vi "VoltageScan.vi"() -> ()   [LabVIEW 2015]
uses:
  Program Files (x86)/National Instruments/LabVIEW 2016/instr.lib/Agilent 428X Series/Agilent 428X Series.lvlib
  Program Files (x86)/National Instruments/LabVIEW 2016/instr.lib/Keithley 24XX/Keithley 24XX.lvlib
  <vilib>/Utility/file.llb/Write Delimited Spreadsheet (string).vi
  <vilib>/Utility/file.llb/Read Delimited Spreadsheet (DBL).vi
  Program Files (x86)/National Instruments/LabVIEW 2016/instr.lib/Keithley 24XX/Public/Data/Read (Single Point).vi
panel:
  in  "Display channel":i32
  out "Data curve for single channel":cluster{"X":dbl[], "Y":dbl[]}[](graph) caption="XY Graph"
  in  "Voltage Limit (V)":dbl=1000.0 format="%#_13g"
  in  "Stop":bool
  in  "Sensor type":enum16{"6''", "8''", "One channel"}(ring)=enum."One channel"
  out "Channels":cluster{i32[], dbl[]}[](graph) caption="XY Graph"
  in  "Voltage Delay (s)":dbl=0.5 format="%#_13g"
  out "Data Status":bool=TRUE
  in  "VISA resource name LCR":refnum<visa-resource-name>
  in  "Compliance  Level (uA)":dbl=10.0
  in  "Enable Voltage Auto Range (T:Enable)":bool=TRUE
  in  "Voltage Manual Range (1.0)":dbl=1.0
  in  "VISA resource name":refnum<visa-resource-name>
  in  "Open after execution?":bool
  out "Output file":path
  in  "Output file":string="test.txt"
  out "Current voltage [V]":dbl
  out "Current channel":i32
  in  "Switch Delay (s)":dbl=0.01 format="%#_13g"
  out "Voltages":cluster{"X":dbl[], "Y":dbl[]}[](graph) caption="XY Graph"
  out "Input file":path
  in  "Measurement type":enum16{"IV", "CV", "Test"}(ring)=enum."Test"
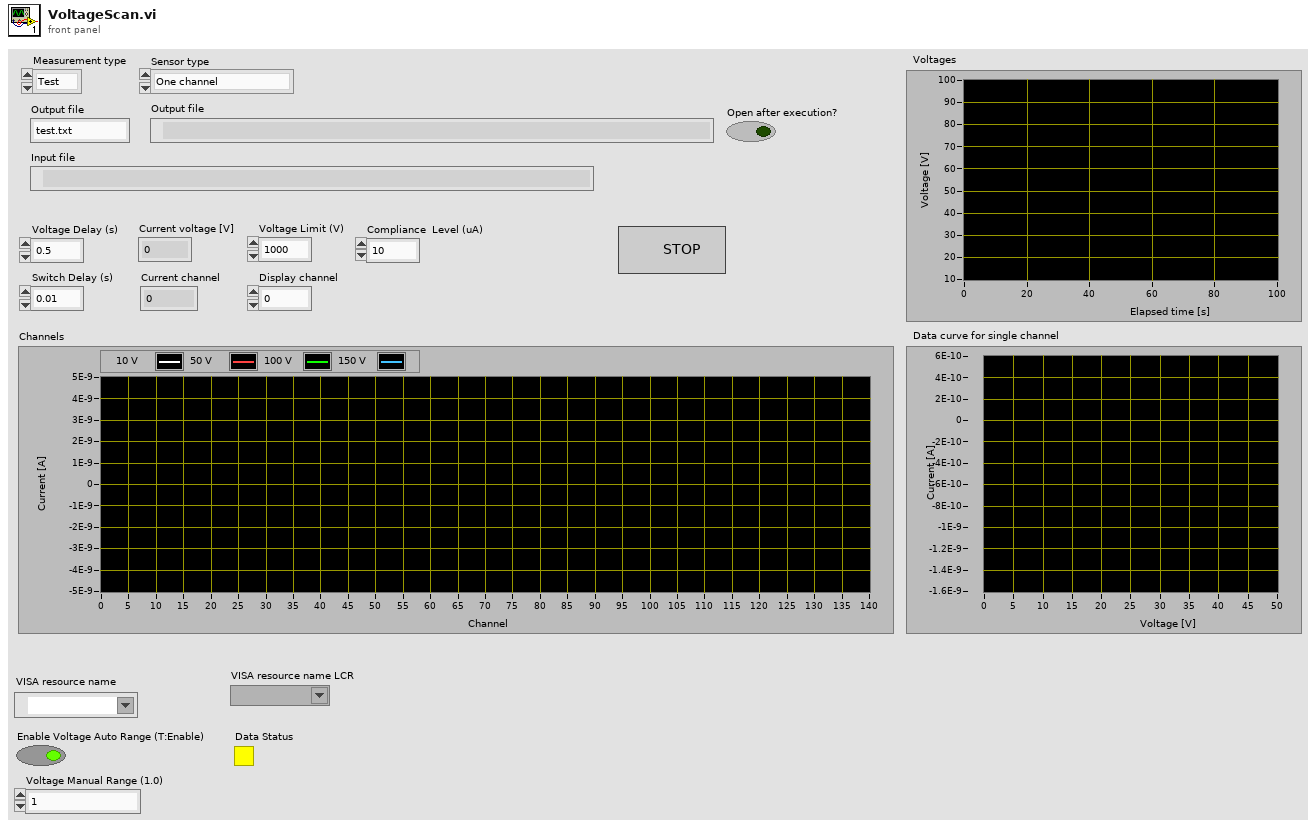
[diagram p1: front panel]
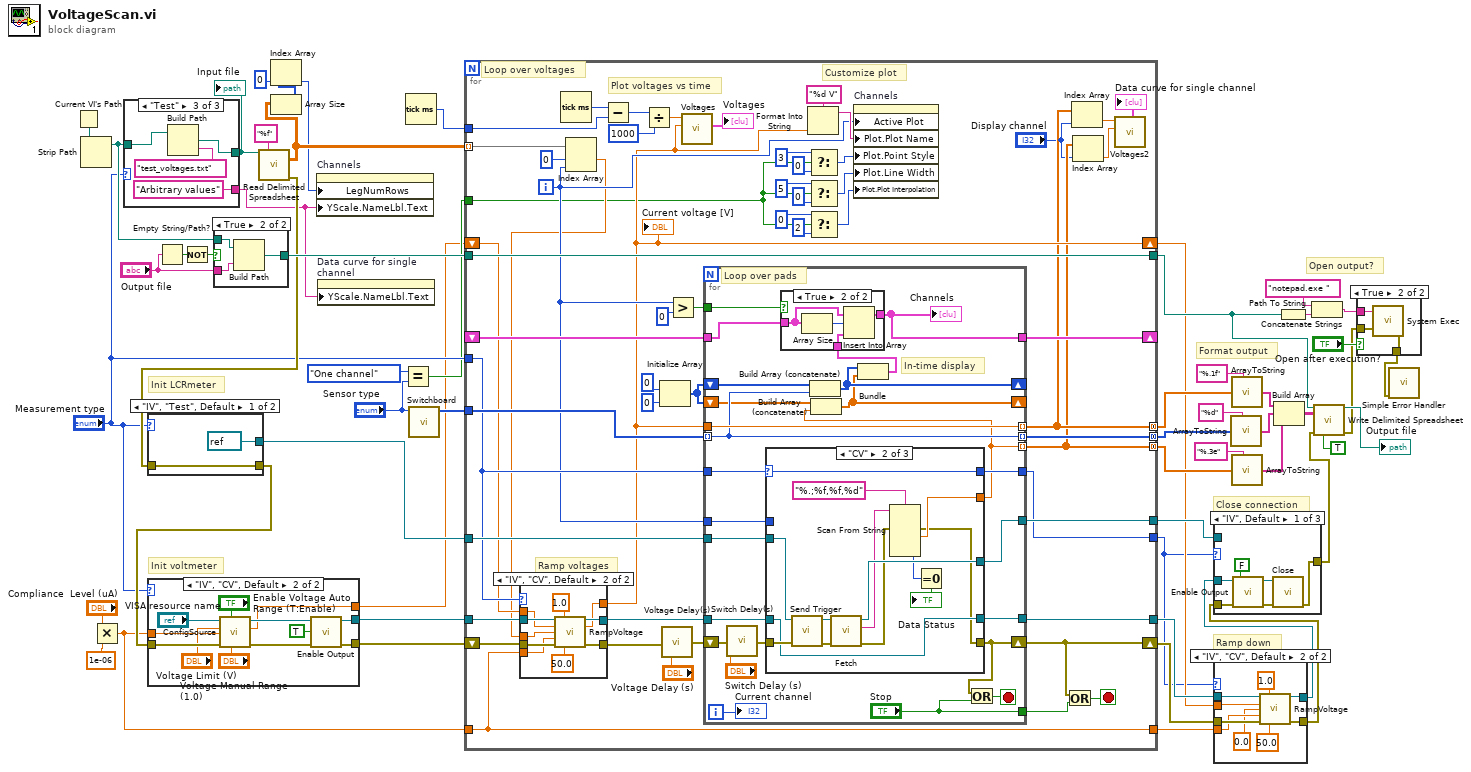
[diagram p0: block diagram]
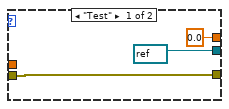
[diagram p3: hidden frame]
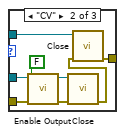
[diagram p4: hidden frame]
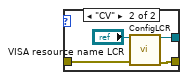
[diagram p6: hidden frame]
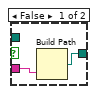
[diagram p8: hidden frame]
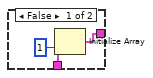
[diagram p10: hidden frame]
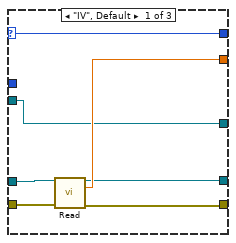
[diagram p11: hidden frame]
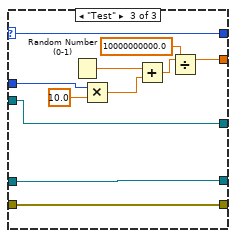
[diagram p12: hidden frame]
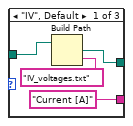
[diagram p13: hidden frame]
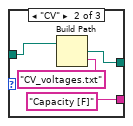
[diagram p14: hidden frame]
diagram:
  # "Close connection"
  # "Ramp down"
  # "Init LCRmeter"
  # "Init voltmeter"
  # "Format output"
  # "Open output?"
  n1 = Current VI's Path() -> (path=w55:path)
  n2 = Strip Path(path=w55) -> (stripped path=w49:path)  [unwired: 1 out]
  n3 = Multiply(x="Compliance  Level (uA)", y=1e-06) -> (x*y=w5:dbl)
  n4 = case shown="\"Test\"" "Measurement type" {
    tunnel: [w58 w62 w66] -> w30
    tunnel: w49 -> [w60 w63 w67]
    tunnel: ["Current [A]" "Capacity [F]" "Arbitrary values"] -> w2
    frame "IV", Default {
      n5 = Build Path(base path=w60, name or relative path="IV_voltages.txt") -> (appended path=w58:path)
    }
    frame "CV" {
      n6 = Build Path(base path=w63, name or relative path="CV_voltages.txt") -> (appended path=w62:path)
    }
    frame "Test" {
      n7 = Build Path(base path=w67, name or relative path="test_voltages.txt") -> (appended path=w66:path)
    }
  }
  "Input file" <- w30
  n8 = Empty String/Path?(string/path="Output file") -> (empty?=w47:bool)
  n9 = Not(x=w47) -> (.not. x?=w45:bool)
  n10 = case shown="True" w45 {
    tunnel: "Output file" -> [w70 w73]
    tunnel: w49 -> [_ w72]
    tunnel: [w69 w71] -> w28
    frame False {
      n11 = Build Path(name or relative path=w70) -> (appended path=w69:path)  [unwired: 1 in]
    }
    frame True {
      n12 = Build Path(base path=w72, name or relative path=w73) -> (appended path=w71:path)
    }
  }
  n13 = call-poly <vilib>:"Read Delimited Spreadsheet.vi"("file path (dialog if empty)"=w30, "format (%.3f)"="%f") -> ("all rows"=w52:dbl[][], "error out"=w24:errorcluster)  [unwired: 8 in, 4 out]
  n14 = case shown="\"IV\", \"Test\", Default" "Measurement type" {
    tunnel: w24 -> [w75 w78]
    tunnel: [w75 w77] -> w23
    tunnel: [refnum<visa-resource-name> refnum ("VISA resource name out") w76] -> w22
    frame "IV", "Test", Default {
    }
    frame "CV" {
      n15 = call "ConfigLCR.vi"("VISA resource name LCR"="VISA resource name LCR", "error in (no error)"=w78) -> ("VISA resource name out"=w76:refnum<visa-resource-name>, "error out"=w77:errorcluster)  [unwired: 12 in]
    }
  }
  n16 = case shown="\"IV\", \"CV\", Default" "Measurement type" {
    tunnel: [refnum<visa-resource-name> refnum ("VISA resource name out") w93] -> w27
    tunnel: [w82 w92] -> w26
    tunnel: w23 -> [w82 w87]
    tunnel: w5 -> [_ w84]
    tunnel: [0.0 ("Output Level (0)") w83] -> w11
    frame "Test" {
    }
    frame "IV", "CV", Default {
      n17 = call "ConfigSource.vi"("Voltage Manual Range (1.0)"="Voltage Manual Range (1.0)", "Single measurement? 2"="Enable Voltage Auto Range (T:Enable)", "error in (no error)"=w87, "Compliance  Level (0.1)"=w84, "Voltage Limit (0.0 V)"="Voltage Limit (V)", "VISA resource name"="VISA resource name") -> ("error out"=w90:errorcluster, "Output Level (0)"=w83:dbl, "VISA resource name out"=w91:refnum<visa-resource-name>)  [unwired: 3 in]
      n18 = call "Enable Output.vi"("error in (no error)"=w90, "Enable Output (T: Enable)"=TRUE ("Enable Output"), "VISA resource name"=w91) -> ("error out"=w92:errorcluster, "VISA resource name out"=w93:refnum<visa-resource-name>)  [unwired: 7 in]
    }
  }
  n19 = Array Size(array=w52) -> (size(s)=w54:i32[])
  n20 = Index Array(array=w54, index=0) -> (element=w17:i32)
  n21 = property on="Channels" class="XYGraph (strict)"("LegNumRows"=w17, "YScale.NameLbl.Text"=w2) -> ()  [unwired: 2 in, 2 out]
  n22 = property on="Data curve for single channel" class="XYGraph (strict)"("YScale.NameLbl.Text"=w2) -> ()  [unwired: 2 in, 2 out]
  n23 = Equal?(x=enum16{"6''", "8''", "One channel"}."One channel" ("Sensor type 2"), y="Sensor type") -> (x = y?=w14:bool)
  n24 = Tick Count (ms)() -> (millisecond timer value=w18:u32)
  n25 = call "Switchboard.vi"("Sensor type"="Sensor type") -> ("Output config"=w51:i32[])  [unwired: 10 in]
  n26 = for {
    tunnel: w52 -> [w149] mode=indexing
    tunnel: w51 -> [w146]
    tunnel: [w101] -> w37 mode=concatenating
    tunnel: [w100] -> w35 mode=concatenating
    tunnel: [w144] -> w36 mode=concatenating
    tunnel: w28 -> [w143]
    tunnel: [w143] -> w25
    tunnel: w27 -> [w142]
    tunnel: [w107] -> w7
    tunnel: "Measurement type" -> [w120]
    shift-right: [w106] -> w8
    shift-left: w26 -> [w139]
    tunnel: w22 -> [w138]
    tunnel: [w134] -> w3
    tunnel: [w140] -> w21
    shift-right: [w132] -> _
    shift-left: _ -> [w131]
    tunnel: w18 -> [w125]
    tunnel: w14 -> [w95]
    tunnel: w5 -> [w104]
    shift-right: [w102] -> w6
    shift-left: w11 -> [w105]
    tunnel: [w104] -> w4
    i -> [w110]
    stop <- w108 stop-if-true
    # "Ramp voltages"
    # "Plot voltages vs time"
    # "Customize plot"
    # "Loop over voltages"
    n27 = Tick Count (ms)() -> (millisecond timer value=w127:u32)
    n28 = Index Array(array=w149, index #1=0 ("index"), index #2=w110) -> (element #1=w103:dbl)  [unwired: 1 out]
    n29 = case shown="\"IV\", \"CV\", Default" w120 {
      tunnel: w142 -> [w152 w159]
      tunnel: w103 -> [w150 w158]
      tunnel: [w152 w161] -> w141
      tunnel: w139 -> [w151 w160]
      tunnel: [w151 w162] -> w136
      tunnel: w104 -> [_ w156]
      tunnel: w105 -> [_ w157]
      tunnel: [w150 w153] -> w102
      frame "Test" {
      }
      frame "IV", "CV", Default {
        n30 = call "RampVoltage.vi"("VISA resource name"=w159, "Delay (s)"=1.0, "Current voltage (V)"=w157, "Target voltage (V)"=w158, "Compliance Current (A)"=w156, "error in (no error)"=w160, "Step size (V)"=50.0) -> ("VISA resource name out"=w161:refnum<visa-resource-name>, "Current voltage out (V)"=w153:dbl, "error out"=w162:errorcluster)  [unwired: 6 in]
      }
    }
    "Current voltage [V]" <- w102
    n31 = Subtract(x=w127, y=w125) -> (x-y=w126:u32)
    n32 = Divide(x=w126, y=u32 1000 ("x")) -> (x/y=w124:dbl)
    n33 = Initialize Array(0 ("dimension size"), 0 ("dimension size")) -> (w128:i32[])
    n34 = call "Voltage Delay(s)"("error in (no error)"=w136, "Delay Time (s)"="Voltage Delay (s)") -> ("error out"=w135:errorcluster)  [unwired: 9 in]
    n35 = Greater?(x=w110, y=0) -> (0:w133:bool)
    n36 = call "Voltages"("Y Input"=w102, "X Input"=w124) -> ("XY Graph"=→"Voltages":cluster{"X":dbl[], "Y":dbl[]}[])  [unwired: 8 in, 1 out]
    n37 = for {
      tunnel: w146 -> [w179] mode=indexing
      tunnel: [w179] -> w144 mode=indexing
      tunnel: [w177] -> w100 mode=indexing
      tunnel: w102 -> [w187]
      tunnel: [w187] -> w101 mode=indexing
      tunnel: w141 -> [w185]
      tunnel: [w184] -> w107
      tunnel: w120 -> [w186]
      shift-right: [w165] -> w106
      shift-left: w135 -> [w166]
      tunnel: w138 -> [w183]
      tunnel: [w182] -> w134
      tunnel: [w181] -> w140
      shift-right: [w175] -> _
      shift-left: w128 -> [w178]
      shift-right: [w174] -> _
      shift-left: w128 -> [w176]
      tunnel: w133 -> [w172]
      tunnel: w110 -> [w173]
      tunnel: w131 -> [w171]
      tunnel: [w169] -> w132
      tunnel: ["Stop"] -> w109
      i -> [w170]
      stop <- w164 stop-if-true
      # "In-time display"
      # "Loop over pads"
      n38 = call "Switch Delay(s)"("error in (no error)"=w166, "Delay Time (s)"="Switch Delay (s)") -> ("error out"=w167:errorcluster)  [unwired: 9 in]
      n39 = case shown="\"CV\"" w186 {
        selector: w186 -> [w196 w212 w226]
        tunnel: [w201 w205 w217] -> w177
        tunnel: w185 -> [w199 w204 w224]
        tunnel: w167 -> [w200 w210 w223]
        tunnel: [w198 w204 w224] -> w184
        tunnel: [w197 w202 w223] -> w165
        tunnel: w183 -> [w195 w213 w225]
        tunnel: [w196 w212 w226] -> w182
        tunnel: [w195 w211 w225] -> w181
        tunnel: w173 -> [_ _ w218]
        frame "IV", Default {
          n40 = call-poly "Read.vi"("VISA resource name"=w199, "error in (no error)"=w200) -> ("VISA resource name out"=w198:refnum<visa-resource-name>, "Current"=w201:sgl, "error out"=w197:errorcluster)  [unwired: 7 in, 4 out]
        }
        frame "CV" {
          n41 = call "Send Trigger.vi"("error in (no error)"=w210, "VISA resource name"=w213) -> ("error out"=w214:errorcluster, "VISA resource name out"=w215:refnum<visa-resource-name>)  [unwired: 8 in]
          n42 = call "Fetch.vi"("error in (no error)"=w214, "VISA resource name"=w215) -> ("error out"=w203:errorcluster, "Returned Data"=w206:string, "VISA resource name out"=w211:refnum<visa-resource-name>)  [unwired: 7 in]
          n43 = Scan From String(format string="%.;%f,%f,%d", input string=w206, error in=w203) -> (error out=w202:errorcluster, output 1=w205:dbl, output 3=w209:i32)  [unwired: 5 in, 2 out]
          n44 = Equal To 0?(x=w209) -> (x = 0?=→"Data Status":bool)
        }
        frame "Test" {
          n45 = Random Number (0-1)() -> (number: 0 to 1=w222:dbl)
          n46 = Multiply(x=w218, y=10.0) -> (x*y=w219:dbl)
          n47 = Add(x=w222, y=w219) -> (x+y=w221:dbl)
          n48 = Divide(x=w221, y=10000000000.0) -> (x/y=w217:dbl)
        }
      }
      n49 = Build Array (concatenate)(w178, w179) -> (w175:i32[])
      n50 = Build Array (concatenate)(w176, w177) -> (w174:dbl[])
      n51 = Bundle(w175, w174) -> (w168:cluster{i32[], dbl[]})  [unwired: 1 out]
      n52 = case shown="True" w172 {
        tunnel: w171 -> [_ w193]
        tunnel: [w188 w192] -> w169
        tunnel: w168 -> [w189 w191]
        frame False {
          n53 = Initialize Array(w189, 1 ("dimension size")) -> (w188:cluster{i32[], dbl[]}[])
        }
        frame True {
          n54 = Array Size(array=w193) -> (size(s)=w194:i32)
          n55 = Insert Into Array(array=w193, index=w194, new element=w191) -> (w192:cluster{i32[], dbl[]}[])
        }
      }
      "Channels" <- w169
      n56 = Or(x=w165, y="Stop") -> (x .or. y?=w164:bool)
      "Current channel" <- w170
    }
    n57 = Format Into String(format string="%d V", w102) -> (resulting string=w122:string)  [unwired: 2 in, 1 out]
    n58 = Select(t=u8 3 ("Plot.Point Style"), s=w95, f=u8 0 ("Plot.Point Style")) -> (s? t:f=w116:u8)
    n59 = Select(t=u8 5 ("Plot.Point Style"), s=w95, f=u8 0 ("Plot.Point Style")) -> (s? t:f=w114:u8)
    n60 = Select(t=u8 0 ("Plot.Point Style"), s=w95, f=u8 2 ("Plot.Point Style")) -> (s? t:f=w111:u8)
    n61 = property on="Channels" class="XYGraph (strict)"("Active Plot"=w110, "Plot.Plot Name"=w122, "Plot.Point Style"=w116, "Plot.Line Width"=w114, "Plot.Plot Interpolation"=w111) -> ()  [unwired: 2 in, 2 out]
    n62 = Or(x=w106, y=w109) -> (x .or. y?=w108:bool)
    n63 = Index Array(array=w101, index="Display channel") -> (element=w97:dbl)
    n64 = Index Array(array=w100, index="Display channel") -> (element=w96:dbl)
    n65 = call "Voltages2"("Y Input"=w96, "X Input"=w97) -> ("XY Graph"=→"Data curve for single channel":cluster{"X":dbl[], "Y":dbl[]}[])  [unwired: 8 in, 1 out]
  }
  n66 = case shown="\"IV\", \"CV\", Default" w3 {
    tunnel: w7 -> [w228 w234]
    tunnel: [w228 w236] -> w9
    tunnel: w8 -> [w227 w235]
    tunnel: [w227 w237] -> w10
    tunnel: w4 -> [_ w232]
    tunnel: w6 -> [_ w233]
    frame "Test" {
    }
    frame "IV", "CV", Default {
      n67 = call "RampVoltage.vi"("VISA resource name"=w234, "Delay (s)"=1.0, "Current voltage (V)"=w233, "Target voltage (V)"=0.0, "Compliance Current (A)"=w232, "error in (no error)"=w235, "Step size (V)"=50.0) -> ("VISA resource name out"=w236:refnum<visa-resource-name>, "error out"=w237:errorcluster)  [unwired: 6 in, 1 out]
    }
  }
  n68 = case shown="\"IV\", Default" w3 {
    tunnel: w21 -> [_ w251 _]
    tunnel: w10 -> [w241 w244 w252]
    tunnel: [w243 w250 w252] -> w20
    tunnel: w9 -> [w240 w245 _]
    frame "IV", Default {
      n69 = call "Enable Output.vi"("error in (no error)"=w241, "Enable Output (T: Enable)"=FALSE ("Enable Output"), "VISA resource name"=w240) -> ("error out"=w238:errorcluster, "VISA resource name out"=w239:refnum<visa-resource-name>)  [unwired: 7 in]
      n70 = call "Close.vi"("error in (no error)"=w238, "VISA resource name"=w239) -> ("error out"=w243:errorcluster)  [unwired: 9 in]
    }
    frame "CV" {
      n71 = call "Enable Output.vi"("error in (no error)"=w244, "Enable Output (T: Enable)"=FALSE ("Enable Output"), "VISA resource name"=w245) -> ("error out"=w246:errorcluster, "VISA resource name out"=w247:refnum<visa-resource-name>)  [unwired: 7 in]
      n72 = call "Close.vi"("error in (no error)"=w246, "VISA resource name"=w247) -> ("error out"=w249:errorcluster)  [unwired: 9 in]
      n73 = call "Close.vi"("error in (no error)"=w249, "VISA resource name"=w251) -> ("error out"=w250:errorcluster)  [unwired: 9 in]
    }
    frame "Test" {
    }
  }
  n74 = call "ArrayToString.vi"("Format"="%d", "Input 1D array"=w36) -> ("Output 1D array"=w39:string[])  [unwired: 7 in]
  n75 = call "ArrayToString.vi"("Format"="%.1f", "Input 1D array"=w37) -> ("Output 1D array"=w40:string[])  [unwired: 7 in]
  n76 = call "ArrayToString.vi"("Format"="%.3e", "Input 1D array"=w35) -> ("Output 1D array"=w41:string[])  [unwired: 7 in]
  n77 = Build Array(w40, w39, w41) -> (w38:string[][])
  n78 = Path To String(path=w25) -> (string=w34:string)
  n79 = Concatenate Strings("notepad.exe " ("string"), w34) -> (w32:string)
  n80 = call-poly <vilib>:"Write Delimited Spreadsheet.vi"("file path (dialog if empty)"=w25, "2D data"=w38, "error in (no error)"=w20, "transpose? (no:F)"=TRUE) -> ("new file path (Not A Path if cancelled)"=→"Output file":path, "error out"=w29:errorcluster)  [unwired: 10 in]
  n81 = case shown="True" "Open after execution?" {
    tunnel: w32 -> [_ w256]
    tunnel: w29 -> [w253 w255]
    tunnel: [w253 w254] -> w1
    frame False {
    }
    frame True {
      n82 = call <vilib>:"System Exec.vi"("error in (no error)"=w255, "command line"=w256) -> ("error out"=w254:errorcluster)  [unwired: 6 in, 3 out]
    }
  }
  n83 = call <vilib>:"Simple Error Handler.vi"("error in (no error)"=w1) -> ()  [unwired: 4 in, 5 out]
